vi "ATS_SetTriggerTimeOut_Brd.vi"(9 "TimeX (1000)":u32=1000, 10 "Timeout (-1s)":dbl=-1.0 format="%.2f", 11 "DeviceIn":i32) -> (0 "Return Code":u32, 2 "Timeout_Set":dbl format="%.2f", 3 "DeviceOut":i32)   [LabVIEW 2015]
doc: "_____AlazarTech, Scope_____\n\nSpecify a timeout for a trigger event for one Board. If no trigger occurs in the specified amount of time, the board automatically forces a trigger.\n\nIf Timeout input is < 0, a Timeout = Clock x Length x TimeX(100) will be used.\n\nMinimum value is 10e-6s.\nMaximum 3600s (1hour)."
uses:
  ATS_ctl/ATS_Global_Ctrl.ctl
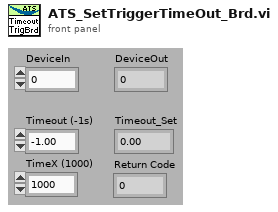
[diagram p1: front panel]
types:
  T1 = typedef "ATS_Global_Ctrl.ctl" = enum16{"Init_Device", "Clear_ALL", "Set", "Get"}
  T2 = typedef "ATS_Set_Value.ctl" = cluster{"Clock (s)":dbl, "RangeA (v)":dbl, "RangeB (v)":dbl, "Ranges (v)":dbl[]}
  T3 = typedef "ATS_Global_4Ch.ctl" = cluster{"Record":T4, "Clock":T5, "Inputs":T9, "Trigger":T15}
  T4 = typedef "Record.ctl" = cluster{"Count":u32, "Presize":u32, "Length":u32}
  T5 = typedef "Clock.ctl" = cluster{"ClckSource":T6, "ClckRate":T7, "ClckEdge":T8, "Decimation":u32}
  T6 = typedef "ClockSource.ctl" = enum16{"Internal", "External", "Medium Ext.", "Slow Ext.", "Ext. AC", "Ext. DC", "Ext. (PLL)"}
  T7 = typedef "ClockRate.ctl" = u32
  T8 = typedef "ClockEdge.ctl" = u16
  T9 = typedef "ATS_InputArray.ctl" = T10[]
  T10 = typedef "InputCtrl.ctl" = cluster{"Coupling":T11, "Range":T12, "Impedance":T13, "Bandwidth":T14}
  T11 = typedef "Coupling.ctl" = enum16{"AC", "DC"}
  T12 = typedef "Range.ctl" = u32
  T13 = typedef "Impedance.ctl" = enum16{"1M ohms", "50 ohms"}
  T14 = typedef "Bandwidth.ctl" = enum16{"Full Bandwidth", "Reduce Bandwidth"}
  T15 = typedef "ATS_Trigger_4Ch.ctl" = cluster{"TrigOperation":T16, "Timeout (s)":dbl, "Trig. Delay":u32, "Engine X":T17, "Engine Y":T17, "ExtTrigControl":T19}
  T16 = typedef "TriggerOperation.ctl" = enum16{"Only X", "Only Y", "X or Y", "X and Y", "X xor Y", "X and not Y", "not X and Y"}
  T17 = typedef "ATS_TriggerEngine_4Ch.ctl" = cluster{"Source":T18, "Slope":enum32{"Positive", "Negative"}, "Level":u32}
  T18 = typedef "ATS_TriggerSource_4Ch.ctl" = enum32{"Chan_A", "Chan_B", "External", "Disable", "Chan_C", "Chan_D"}
  T19 = typedef "ExtTrigger.ctl" = cluster{"Coupling":T11, "Range":T20}
  T20 = typedef "ExtTrigRange.ctl" = enum16{"1 V", "5 V", "TTL"}
  T21 = typedef "Device_Info.ctl" = cluster{"Handle":u32, "Board":string, "CPLD":string, "MemorySize":u32, "SampleSize":u8, "ID":i32, "High_Memory":bool, "Chan/Board":u8}
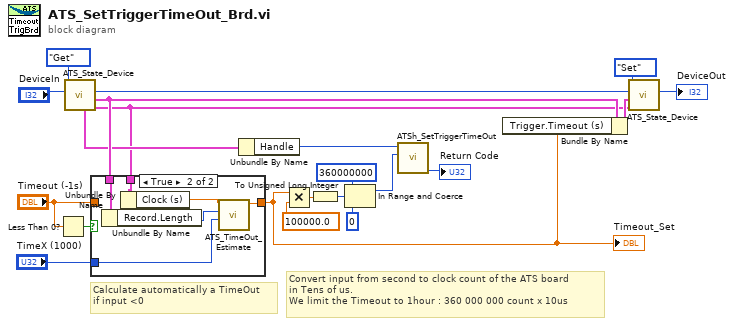
[diagram p0: block diagram]
diagram:
  # "Calculate automatically a TimeOut\nif input <0"
  # "Convert input from second to clock count of the ATS board\nin Tens of us.\nWe limit the Timeout to 1hour : 360 000 000 count x 10us"
  n1 = Less Than 0?(x="Timeout (-1s)") -> (x < 0?=w5:bool)
  n2 = call "ATS_State_Device.vi"("DeviceIn"="DeviceIn", "ATS_GBL_Ctrl"=ATS_Global_Ctrl."Get") -> ("Ref_Out"=w2:T2, "SetupOut"=w8:T3, "DeviceOut"=w10:i32, "DevInfo_Out"=w3:T21)  [unwired: 4 in, 2 out]
  n3 = case shown="True" w5 {
    tunnel: w8 -> [_ w28]
    tunnel: "TimeX (1000)" -> [_ w26]
    tunnel: "Timeout (-1s)" -> [w22 _]
    tunnel: [w22 w25] -> w6
    tunnel: w2 -> [_ w24]
    frame False {
    }
    frame True {
      n4 = Unbundle By Name(w28) -> ("Record.Length"=w27:u32)
      n5 = Unbundle By Name(w24) -> ("Clock (s)"=w23:dbl)
      n6 = call "ATS_TimeOut_Estimate.vi"("Mult (20)"=w26, "Rec.Length (B)"=w27, "Clock_Value"=w23) -> ("TimeOut"=w25:dbl)  [unwired: 4 in]
    }
  }
  "Timeout_Set" <- w6
  n7 = Unbundle By Name(w3) -> ("Handle"=w11:u32)
  n8 = Multiply(x=w6, y=100000.0) -> (x*y=w18:dbl)
  n9 = To Unsigned Long Integer(number=w18) -> (unsigned 32bit integer=w17:u32)
  n10 = In Range and Coerce(upper limit=u32 360000000, x=w17, lower limit=u32 0) -> (coerced(x)=w16:u32)  [unwired: 1 out]
  n11 = call "ATSh_SetTriggerTimeOut.vi"("TimeoutCount"=w16, "Handle"=w11) -> ("Return Code"=→"Return Code":u32)  [unwired: 8 in, 1 out]
  n12 = Bundle By Name(cluster=w8, "Trigger.Timeout (s)"=w6) -> (w14:T3)
  n13 = call "ATS_State_Device.vi"("Ref_In"=w2, "SetupIn"=w14, "DeviceIn"=w10, "ATS_GBL_Ctrl"=ATS_Global_Ctrl."Set") -> ("DeviceOut"=→"DeviceOut":i32)  [unwired: 2 in, 5 out]
